vi "Test VI Window Icon.vi"   [LabVIEW 2023]
uses:
  Glyph/VI Icon Canvas/VI Icon Canvas.lvclass
  Canvas/Drawer .Net.lvclass
  LV-Awesome/LV Awesome/LV Awesome.lvclass
types:
  T1 = cluster{"Front":cluster{"Color":u32, "Alpha":u8}, "Back":cluster{"Color":u32, "Alpha":u8}}
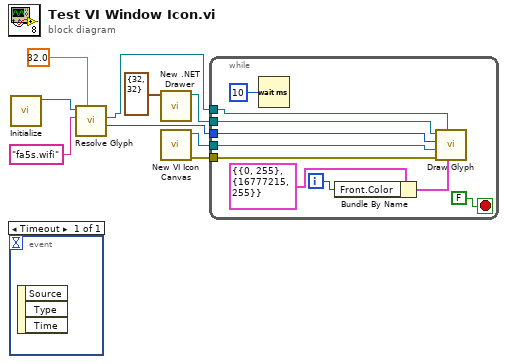
[diagram p0: block diagram]
diagram:
  n1 = event shown="[0] Timeout" {
    selector: _ -> [_]
    dyn-events: _ -> [_]
    timeout: _ -> [_]
    event Timeout {
      n2 = event-data() -> ()  [unwired: 1 in, 3 out]
    }
  }
  n3 = call "Initialize.vi"() -> ("LV Awesome"=w5:refnum<class "LV Awesome.lvclass">)  [unwired: 10 in, 1 out]
  n4 = call-dynamic "Resolve Glyph.vi"("Size"=32.0, "Glyph Name"="fa5s.wifi", "LV-Awesome.lvlib:LV Awesome.lvclass"=w5) -> ("charcode"=w3:u32, "Font Settings out"=w2:refnum<class "Font Settings.lvclass">)  [unwired: 5 in, 2 out]
  n5 = call "New .NET Drawer.vi"("Size"=cluster{"width":i32, "height":i32} {"width"=32, "height"=32}) -> ("Canvas out"=w6:refnum<class "Drawer .Net.lvclass">)  [unwired: 9 in, 1 out]
  n6 = call "New VI Icon Canvas.vi"() -> ("error out"=w8:errorcluster, "VI Icon Canvas out"=w9:refnum<class "VI Icon Canvas.lvclass">)  [unwired: 10 in]
  n7 = while {
    tunnel: w9 -> [w19]
    tunnel: w8 -> [w18]
    tunnel: w6 -> [w17]
    tunnel: w3 -> [w16]
    tunnel: w2 -> [w15]
    i -> [w12]
    stop <- FALSE stop-if-true
    n8 = Wait (ms)(milliseconds to wait=u32 10) -> ()  [unwired: 1 out]
    n9 = Bundle By Name(cluster=T1 {"Front"={"Color"=0, "Alpha"=255}, "Back"={"Color"=16777215, "Alpha"=255}} ("Colors"), "Front.Color"=w12) -> (w13:T1)
    n10 = call-dynamic "Draw Glyph.vi"("Colors"=w13, "Font (System)"=w15, "error in (no error)"=w18, "Destination"=w19, "codepoint"=w16, "Canvas .Net in"=w17) -> ()  [unwired: 3 in, 3 out]
  }
